vi "SaveLog.vi"(8 "错误输入（无错误）":errorcluster, 11 "AllControls In":T1) -> (0 "错误输出":errorcluster)   [LabVIEW 2017]
uses:
  Ctrls/AllControls.ctl
  Ctrls/PathChoose.ctl
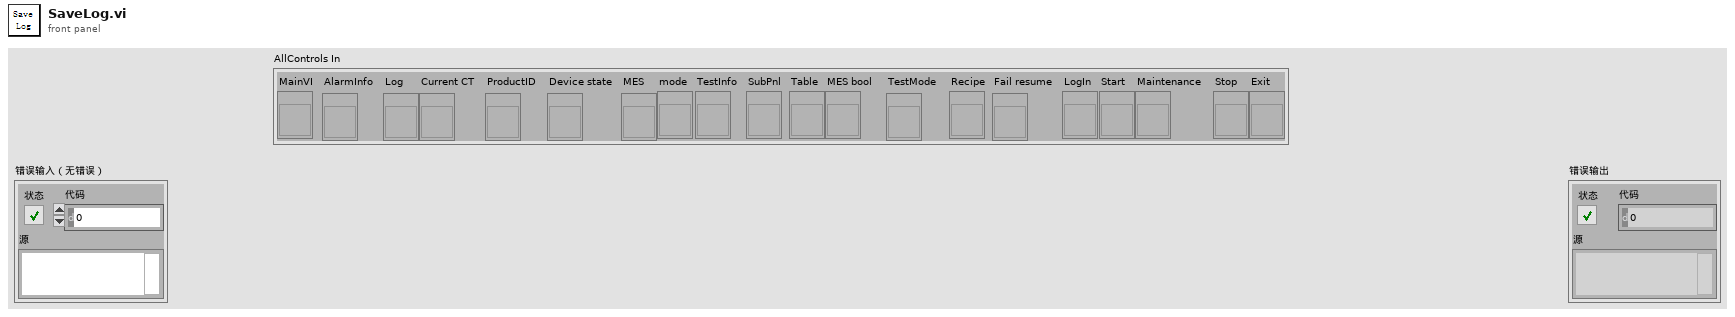
[diagram p1: front panel]
types:
  T1 = typedef "AllControls.ctl" = cluster{"MainVI":refnum<vi>, "AlarmInfo":refnum<vi>, "Log":refnum<vi>, "Current CT":refnum<vi>, "ProductID":refnum<vi>, "Device state":refnum<vi>, "MES":refnum<vi>, "mode":refnum<vi>, "TestInfo":refnum<vi>, "SubPnl":refnum<vi>, "Table":refnum<vi>, "MES bool":refnum<vi>, "TestMode":refnum<vi>, "Recipe":refnum<vi>, "Fail resume":refnum<vi>, "LogIn":refnum<vi>, "Start":refnum<vi>, "Maintenance":refnum<vi>, "Stop":refnum<vi>, "Exit":refnum<vi>}
  T2 = typedef "amc_Message Queue.ctl" = refnum<queue>
  T3 = typedef "PathChoose.ctl" = enum16{"OperatorLog", "AutoRunLog", "AlmLog", "TestData", "AllTestData", "backup_nvm", "backup_before_flashing"}
  T4 = enum16{"open", "replace", "create", "open or create", "replace or create", "replace or create with confirmation"}
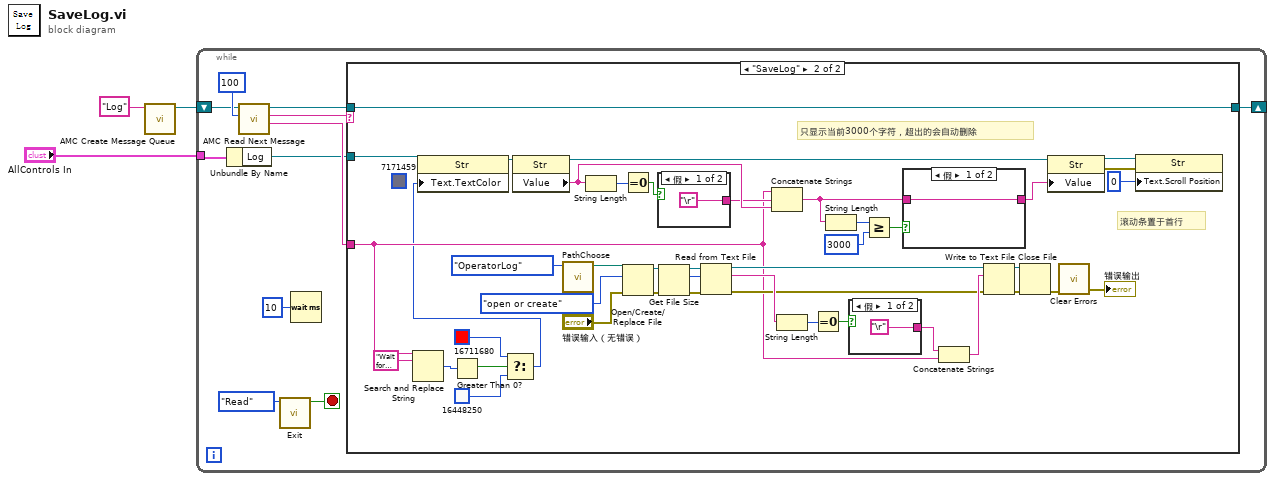
[diagram p0: block diagram]
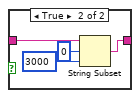
[diagram p3: hidden frame]
diagram:
  n1 = call "AMC Create Message Queue.vi"("Message Queue Name"="Log" ("Message queue name (unnamed)")) -> ("Message Queue out"=w3:T2)  [unwired: 4 in, 6 out]
  n2 = while {
    shift-right: [w10] -> _
    shift-left: w3 -> [w12]
    tunnel: "AllControls In" -> [w8]
    stop <- w5 stop-if-true
    n3 = Unbundle By Name(w8) -> ("Log"=w6:refnum<vi>)
    n4 = call "AMC Read Next Message.vi"("timeout (1ms)"=100 ("Timeout"), "Message Queue in"=w12) -> ("Message Value"=w7:string, "Message Name"=w11:string, "Message Queue out"=w9:T2)  [unwired: 2 in, 5 out]
    n5 = call "Exit.vi"("Step"=enum16{"Initial", "Write", "Read"}."Read" ("step")) -> ("Exit Out"=w5:bool)  [unwired: 9 in, 1 out]
    n6 = Wait (ms)(milliseconds to wait=u32 10) -> ()  [unwired: 1 out]
    n7 = case shown="\"SaveLog\"" w11 {
      tunnel: [w15 w58] -> w10
      tunnel: w9 -> [w15 w58]
      tunnel: w7 -> [_ w22]
      tunnel: w6 -> [_ w23]
      frame "假", Default {
      }
      frame "SaveLog" {
        (unwired) u32 7171459 ("TextColor")
        # "只显示当前3000个字符，超出的会自动删除"
        # "滚动条置于首行"
        n8 = Search and Replace String(input string=w22, search string="Wait for PLC reset single") -> (number of replacements=w20:i32)  [unwired: 6 in, 3 out]
        n9 = Greater Than 0?(x=w20) -> (x > 0?=w19:bool)
        n10 = Select(t=u32 16711680 ("TextColor"), s=w19, f=u32 16448250 ("TextColor")) -> (s? t:f=w17:u32)
        n11 = property class="Str"(reference=w23, "Text.TextColor"=w17) -> (reference out=w56:refnum<vi>)  [unwired: 1 in, 1 out]
        n12 = property class="Str"(reference=w56) -> (reference out=w29:refnum<vi>, "Value"=w47:string)  [unwired: 1 in, 1 out]
        n13 = call "PathChoose.vi"(11:PathChoose."OperatorLog") -> ("Path_Out"=w46:path)  [unwired: 10 in]
        n14 = String Length(string=w47) -> (length=w28:i32)
        n15 = Equal To 0?(x=w28) -> (x = 0?=w30:bool)
        n16 = Open/Create/Replace File(file path (use dialog)=w46, error in="错误输入（无错误）", operation (0:open)=T4."open or create" ("操作(0:open)")) -> (refnum out=w32:refnum<file>, error out=w33:errorcluster)  [unwired: 3 in, 1 out]
        n17 = case shown="假" w30 {
          tunnel: ["\r" _] -> w31
          frame False {
          }
          frame True {
          }
        }
        n18 = Get File Size ("获取文件大小")(file=w32, error in=w33) -> (refnum out=w34:refnum<file>, size (in bytes)=w36:i64, 0:w35:errorcluster)
        n19 = Read from Text File ("读取文本文件")(file (use dialog)=w34, count=w36, error in=w35) -> (refnum out=w37:refnum<file>, text=w41:string, error out=w38:errorcluster)  [unwired: 1 in, 1 out]
        n20 = Concatenate Strings(w22, w31, w47) -> (w52:string)
        n21 = String Length(string=w41) -> (length=w40:i32)
        n22 = Equal To 0?(x=w40) -> (x = 0?=w39:bool)
        n23 = String Length(string=w52) -> (length=w50:i32)
        n24 = case shown="假" w39 {
          tunnel: ["\r" _] -> w42
          frame False {
          }
          frame True {
          }
        }
        n25 = Greater Or Equal?(x=w50, y=3000) -> (x >= y?=w51:bool)
        n26 = case shown="假" w51 {
          tunnel: w52 -> [w59 w63]
          tunnel: [w59 w60] -> w53
          frame False {
          }
          frame True {
            n27 = String Subset(string=w63, offset (0)=0 ("偏移量(0)"), length (rest)=3000 ("长度（剩余）")) -> (substring=w60:string)
          }
        }
        n28 = Concatenate Strings(w42, w22) -> (w43:string)
        n29 = Write to Text File ("写入文本文件")(file (use dialog)=w37, text=w43, error in=w38) -> (refnum out=w44:refnum<file>, error out=w45:errorcluster)  [unwired: 1 in, 1 out]
        n30 = Close File(refnum=w44, error in=w45) -> (error out=w49:errorcluster)  [unwired: 1 out]
        n31 = property class="Str"(reference=w29, "Value"=w53) -> (reference out=w54:refnum<vi>, error out=w55:errorcluster)  [unwired: 1 in]
        n32 = call <vilib>:"Clear Errors.vi"("error in (no error)"=w49) -> ("error out"=→"错误输出":errorcluster)  [unwired: 5 in, 1 out]
        n33 = property class="Str"(reference=w54, error in=w55, "Text.Scroll Position"=u32 0 ("文本.滚动条位置")) -> ()  [unwired: 2 out]
      }
    }
  }
